vi "Delay Recall.vi"(7 "Channel  (1: CH1)":u16(ring)=1 items=["CH1"=1, "CH2"=2], 8 "error in (no error)":errorcluster, 10 "Number(0~9)":u8 max=9, 11 "VISA resource name":refnum<visa-resource-name>) -> (0 "error out":errorcluster, 3 "VISA resource name out":refnum<visa-resource-name>)   [LabVIEW 2020, in "GPP.lvlib"]
uses:
  GPP.lvlib
  Function/VISA_COMMON.ctl
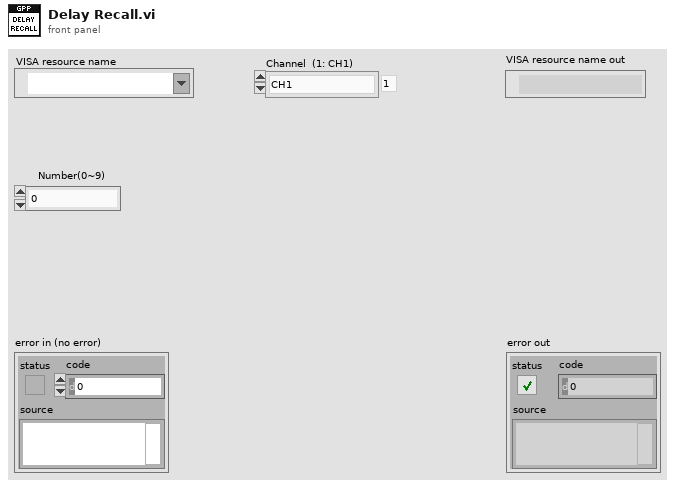
[diagram p1: front panel]
types:
  T1 = typedef "GPP.lvlib/VISA_COMMON.ctl" = enum16{"Initial", "Write CMD", "Read Result", "Read History", "Close"}
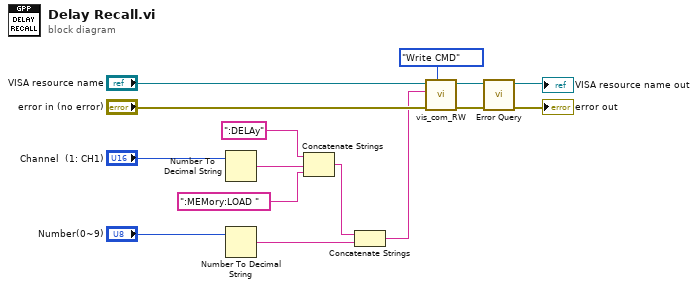
[diagram p0: block diagram]
diagram:
  n1 = Number To Decimal String(number="Channel  (1: CH1)") -> (decimal integer string=w12:string)  [unwired: 1 in]
  n2 = Number To Decimal String(number="Number(0~9)") -> (decimal integer string=w8:string)  [unwired: 1 in]
  n3 = Concatenate Strings(":DELAy", w12, ":MEMory:LOAD ") -> (w14:string)
  n4 = Concatenate Strings(w14, w8) -> (w2:string)
  n5 = call "vis_com_RW.vi"("Funciton"=VISA_COMMON."Write CMD", "error in (no error)"="error in (no error)", "CMD String"=w2, "VISA resource in"="VISA resource name") -> ("error out"=w5:errorcluster, "VISA resource out"=w6:refnum<visa-resource-name>)  [unwired: 5 in, 1 out]
  n6 = call "Error Query.vi"("error in (no error)"=w5, "VISA resource name"=w6) -> ("error out"=→"error out":errorcluster, "VISA resource name out"=→"VISA resource name out":refnum<visa-resource-name>)  [unwired: 6 in, 2 out]
